vi "getAll.vi"(8 "error in (no error)":errorcluster, 11 "Instrument in":refnum<class "Instrument.lvclass">) -> (0 "error out":errorcluster, 1 "getAll":variant, 3 "Instrument out":refnum<class "Instrument.lvclass">)   [LabVIEW 2019, in "Instrument.lvlib" / "Instrument.lvclass"]
doc: "Send \"getAll\" command to remote Instrument. Returns contents of \"getAll.ctl\""
uses:
  Instrument.lvclass
  Typedefs/Instrument.Commands--Enum.ctl
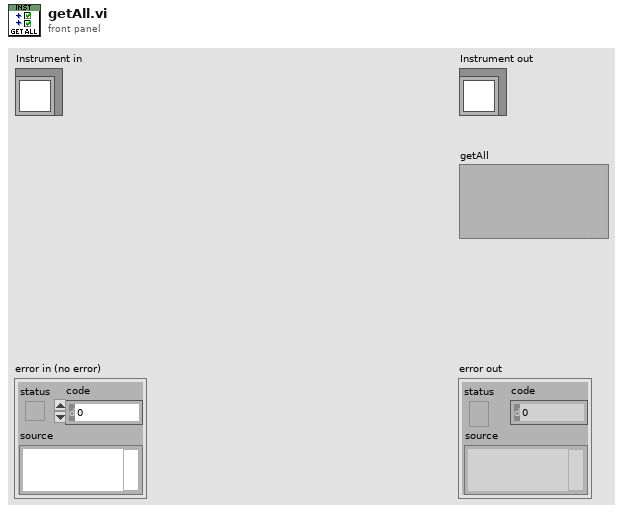
[diagram p1: front panel]
types:
  T1 = typedef "Instrument.lvlib/Instrument.lvclass/Instrument.Commands--Enum.ctl" = enum16{"ACK", "HELP", "IDN", "getAll", "getAllData"}
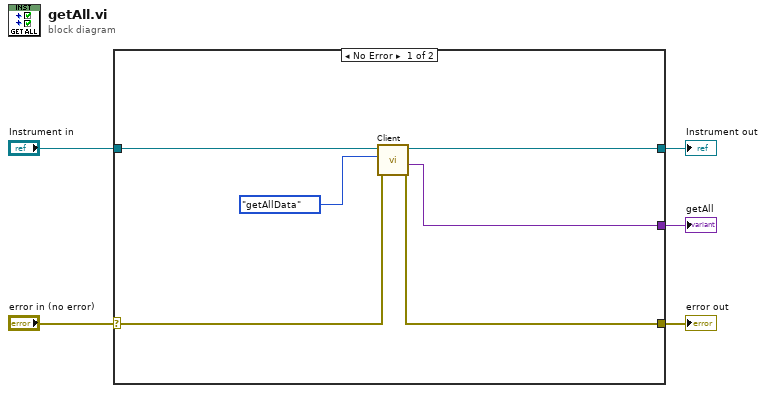
[diagram p0: block diagram]
diagram:
  n1 = case shown="No Error" "error in (no error)" {
    selector: "error in (no error)" -> [w9 w13]
    tunnel: [w6 w13] -> w4
    tunnel: [w8 w12] -> w2
    tunnel: "Instrument in" -> [w11 w12]
    tunnel: [w7 _] -> w1
    frame No Error {
      n2 = call-dynamic "Client.vi"("error in (no error)"=w9, "Command in"=Instrument.Commands--Enum."getAllData" ("Commands"), "Instrument in"=w11) -> ("error out"=w6:errorcluster, "Data out"=w7:variant, "Instrument out"=w8:refnum<class "Instrument.lvclass">)  [unwired: 5 in, 1 out]
    }
    frame Error {
    }
  }
  "error out" <- w4
  "Instrument out" <- w2
  "getAll" <- w1
